vi "Read Ratiometer file.vi"() -> ()   [LabVIEW 2013]
uses:
  JSONtext.lvlib
panel:
  out "error out":errorcluster
  out "text":string
  out "Found":bool
  out "Array":string[](array[string])
  out "<JSON>":string caption="JSON substring"
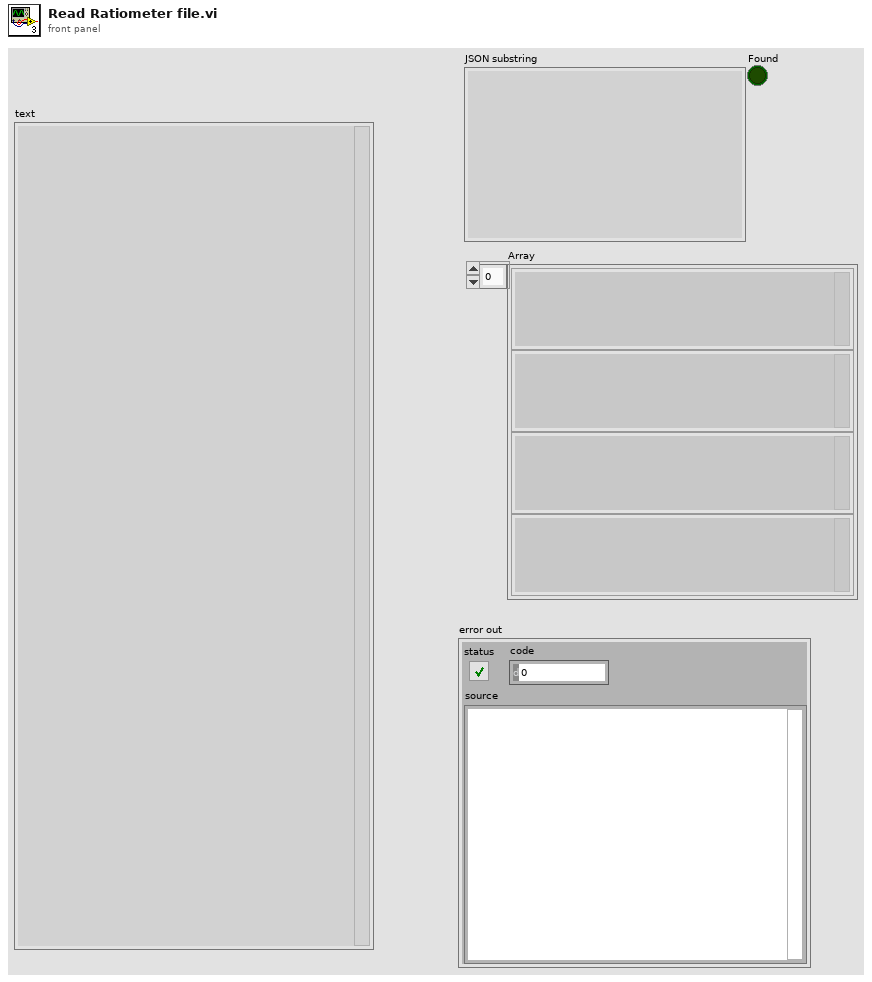
[diagram p1: front panel]
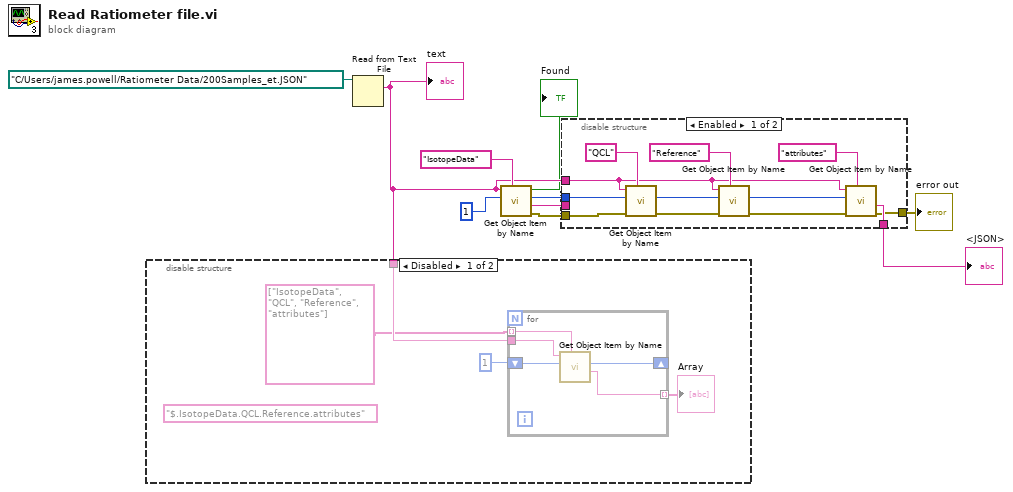
[diagram p0: block diagram]
diagram:
  n1 = Read from Text File(file (use dialog)=path "C:/Users/james.powell/Ratiometer Data/200Samples_et.JSON") -> (text=w5:string)  [unwired: 3 in, 3 out]
  "text" <- w5
  n2 = disable-structure shown="Disabled" {
    disable-tunnel: w5 -> [w13 _]
    frame Disabled {
      (unwired) "$.IsotopeData.QCL.Reference.attributes" ("Item Name")
      n3 = for {
        shift-right: [w19] -> _
        shift-left: 1 ("Object Offset") -> [w18]
        tunnel: w13 -> [w17]
        tunnel: [w16] -> w12 mode=indexing
        tunnel: string[] ["IsotopeData", "QCL", "Reference", "attributes"] -> [w15] mode=indexing
        n4 = call "Get Object Item by Name.vi"("Item Name"=w15, "Object Offset"=w18, "JSON"=w17) -> ("<JSON>"=w16:string, "Item Offset (-1 if not found)"=w19:i32)  [unwired: 5 in, 2 out]
      }
      "Array" <- w12
    }
    frame Enabled {
    }
  }
  n5 = call "Get Object Item by Name.vi"("Item Name"="IsotopeData", "Object Offset"=1, "JSON"=w5) -> ("error out"=w2:errorcluster, "<JSON>"=w4:string, "Item Offset (-1 if not found)"=w7:i32, "Found"=→"Found":bool)  [unwired: 5 in]
  n6 = disable-structure shown="Enabled" {
    disable-tunnel: w7 -> [w30 _]
    disable-tunnel: [w25 w33] -> w6
    disable-tunnel: w5 -> [w24 _]
    disable-tunnel: w4 -> [_ w33]
    disable-tunnel: w2 -> [w23 w32]
    disable-tunnel: [w20 w32] -> w1
    frame Enabled {
      n7 = call "Get Object Item by Name.vi"("Item Name"="QCL", "error in (no error)"=w23, "Object Offset"=w30, "JSON"=w24) -> ("error out"=w22:errorcluster, "Item Offset (-1 if not found)"=w28:i32)  [unwired: 4 in, 2 out]
      n8 = call "Get Object Item by Name.vi"("Item Name"="Reference", "error in (no error)"=w22, "Object Offset"=w28, "JSON"=w24) -> ("error out"=w21:errorcluster, "Item Offset (-1 if not found)"=w26:i32)  [unwired: 4 in, 2 out]
      n9 = call "Get Object Item by Name.vi"("Item Name"="attributes", "error in (no error)"=w21, "Object Offset"=w26, "JSON"=w24) -> ("error out"=w20:errorcluster, "<JSON>"=w25:string)  [unwired: 4 in, 2 out]
    }
    frame Disabled {
    }
  }
  "<JSON>" <- w6
  "error out" <- w1
